vi "Toggle.vi"(11 "Input":bool) -> (2 "output":bool)   [LabVIEW 2015]
uses:
  <vilib>/ptbypt/NI_PtbyPt.lvlib
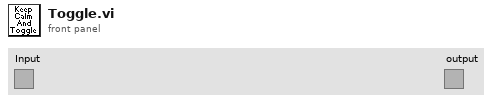
[diagram p1: front panel]
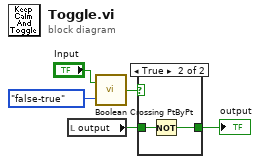
[diagram p0: block diagram]
diagram:
  n1 = local read "output"() -> (w1:bool)
  n2 = call <vilib>:"Boolean Crossing PtByPt.vi"("direction"=enum16{"either", "false-true", "true-false"}."false-true", "input"="Input") -> ("crossing"=w4:bool)  [unwired: 1 in]
  n3 = case shown="True" w4 {
    tunnel: [w6 w8] -> w2
    tunnel: w1 -> [w6 w7]
    frame False {
    }
    frame True {
      n4 = Not(x=w7) -> (.not. x?=w8:bool)
    }
  }
  "output" <- w2
